vi "Read High Time.vi"(8 "error in (no error)":errorcluster, 11 "Servo Switch in":refnum<class "Servo Switch.lvclass">) -> (0 "error out":errorcluster, 2 "High Time":u32, 3 "Servo Switch out":refnum<class "Servo Switch.lvclass">)   [LabVIEW 2019, in "Servo Switch.lvclass"]
uses:
  Servo Switch.lvclass
  Servo Switch.lvclass/Servo Switch.ctl
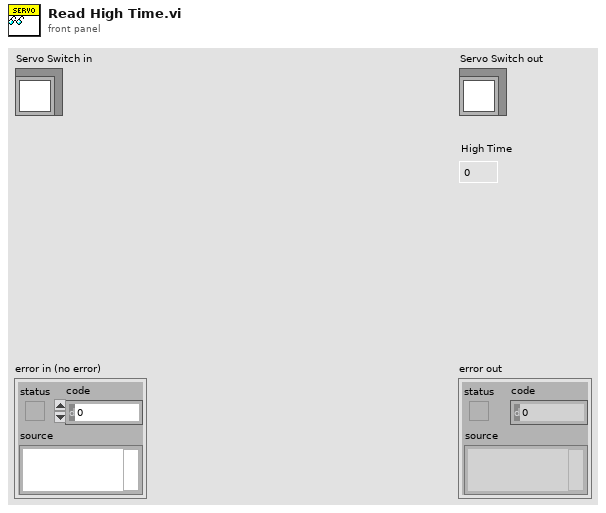
[diagram p1: front panel]
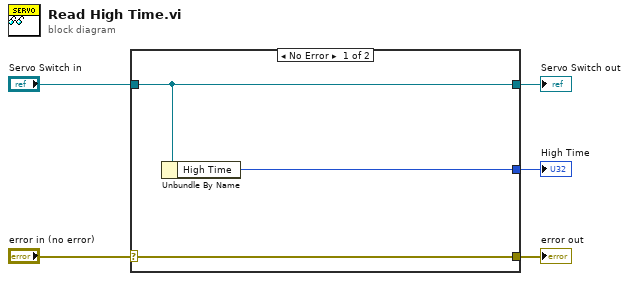
[diagram p0: block diagram]
diagram:
  n1 = case shown="No Error" "error in (no error)" {
    selector: "error in (no error)" -> [w8 w9]
    tunnel: [w8 w9] -> w4
    tunnel: [w7 w10] -> w2
    tunnel: "Servo Switch in" -> [w7 w10]
    tunnel: [w6 _] -> w1
    frame No Error {
      n2 = Unbundle By Name(w7) -> ("High Time"=w6:u32)
    }
    frame Error {
    }
  }
  "error out" <- w4
  "Servo Switch out" <- w2
  "High Time" <- w1
